vi "_SparkGetStatus.vi"(11 "SparkStatus":string="<SparkStatus>\n  <Autosampler>\n    <DeviceStatus>Standby</DeviceStatus>\n    <Detected>\n      <CanMixAndDilute>true</CanMixAndDilute>\n      <SerialNumber>000000</SerialNumber>\n      <FirmwareVersion>1.30</FirmwareVersion>\n      <PcbPartNumber>0840.604-03</PcbPartNumber>\n      <FpgaPartNumber>0840.141</FpgaPartNumber>\n      <FpgaVersion>2.10</FpgaVersion>\n      <FirmwarePartNumber>0840.100</FirmwarePartNumber>\n    </Detected>\n    <DetailedStatus>\n      <ActualTemperature>35</ActualTemperature>\n      <Setpoint>4</Setpoint>\n      <SamplePosition>NotAvailable</SamplePosition>\n      <Status>Standby</Status>\n      <InjectorPosition>Inject</InjectorPosition>\n      <IsVialMissing>false</IsVialMissing>\n      <PlatePosition>NotAvailable</PlatePosition>\n      <IsTemperatureControlOn>false</IsTemperatureControlOn>\n      <StatusCode>0</StatusCode>\n      <ErrorCode>0</ErrorCode>\n      <LastDCActionGuid>00000000-0000-0000-0000-000000000000</LastDCActionGuid>\n      <DoorOpenTime>0</DoorOpenTime>\n      <CommunicationErrorMessage />\n      <IsDoorOpen>false</IsDoorOpen>\n      <TrayType>Vials48</TrayType>\n      <Progress>0</Progress>\n    </DetailedStatus>\n    <LogCounters>\n      <InjectorValve>466</InjectorValve>\n      <IssA>0</IssA>\n      <SyringeValve>2569</SyringeValve>\n      <Syringe>3837</Syringe>\n    </LogCounters>\n    <AdvancedStatus>\n      <IssValvePosition>OneTwo</IssValvePosition>\n      <Valve1Out6Position>0</Valve1Out6Position>\n      <SSVPosition>Solvent1</SSVPosition>\n      <IsCompressorOn>false</IsCompressorOn>\n      <SyringeValvePosition>0</SyringeValvePosition>\n      <AdjustmentNeedleHorizontal>0</AdjustmentNeedleHorizontal>\n      <AdjustmentTray>0</AdjustmentTray>\n      <AdjustmentSyringe>0</AdjustmentSyringe>\n      <AdjustmentNeedleInEEprom>0</AdjustmentNeedleInEEprom>\n      <AdjustmentTrayInEEprom>0</AdjustmentTrayInEEprom>\n      <AdjustmentSyringeInEEprom>0</AdjustmentSyringeInEEprom>\n      <IsAux1On>false</IsAux1On>\n    </AdvancedStatus>\n    <Options>\n      <HasCooling>true</HasCooling>\n      <HasSSV>true</HasSSV>\n      <HasWashPort2>true</HasWashPort2>\n      <HasISSA>false</HasISSA>\n      <HasHeating>false</HasHeating>\n      <Has6PortValve>false</Has6PortValve>\n    </Options>\n    <Config>\n      <LoopVolume>100</LoopVolume>\n      <SyringeVolume>500</SyringeVolume>\n      <NeedleVolume>15</NeedleVolume>\n    </Config>\n  </Autosampler>\n  <ColumnOven>\n    <DeviceStatus>Standby</DeviceStatus>\n    <Detected>\n      <SerialNumber>130086</SerialNumber>\n      <FirmwareVersion>3.01</FirmwareVersion>\n      <PcbPartNumber>0886.603</PcbPartNumber>\n      <FpgaPartNumber>0886.104</FpgaPartNumber>\n      <FpgaVersion>1.00</FpgaVersion>\n      <FirmwarePartNumber>0886.105</FirmwarePartNumber>\n      <PcbVersion>03</PcbVersion>\n      <ColumnOvenOptions>\n        <HasCooling>false</HasCooling>\n        <HasColumnSwitcher>false</HasColumnSwitcher>\n      </ColumnOvenOptions>\n    </Detected>\n    <DetailedStatus>\n      <Status>Standby</Status>\n      <Setpoint>40</Setpoint>\n      <ActualTemperature>36</ActualTemperature>\n      <ActualValvePosition>0</ActualValvePosition>\n      <VapourAlarmSensitivity>Standard</VapourAlarmSensitivity>\n      <StatusCode>0</StatusCode>\n      <ErrorCode>0</ErrorCode>\n      <LastDCActionGuid>00000000-0000-0000-0000-000000000000</LastDCActionGuid>\n      <RequestSetpoint>0</RequestSetpoint>\n      <CustomCommandResponse />\n      <IsOvenOn>false</IsOvenOn>\n    </DetailedStatus>\n    <Service>\n      <IsInServiceMode>false</IsInServiceMode>\n      <ColumnSelectionHomeSensor>Unknown</ColumnSelectionHomeSensor>\n      <ColumnSelectionLegalSensor>Unknown</ColumnSelectionLegalSensor>\n      <HeaterFanSpeed>0</HeaterFanSpeed>\n    </Service>\n    <LogCounters>\n      <ColumnSwitch>0</ColumnSwitch>\n    </LogCounters>\n    <FlashStatus>\n      <Status>Ready</Status>\n      <StatusOfFlash>0</StatusOfFlash>\n      <Percentage>0</Percentage>\n      <Speed>0</Speed>\n    </FlashStatus>\n  </ColumnOven>\n  <LcPump>\n    <DeviceStatus>Running</DeviceStatus>\n    <DetectedA>\n      <SerialNumber>130060</SerialNumber>\n      <FirmwareVersion>1.14</FirmwareVersion>\n      <PcbPartNumber>0760.600-12</PcbPartNumber>\n      <FpgaPartNumber>0760.101</FpgaPartNumber>\n      <FpgaVersion>1.05</FpgaVersion>\n      <FirmwarePartNumber>0760.100</FirmwarePartNumber>\n    </DetectedA>\n    <DetectedB>\n      <SerialNumber>130060</SerialNumber>\n      <FirmwareVersion>1.14</FirmwareVersion>\n      <PcbPartNumber>0760.600-12</PcbPartNumber>\n      <FpgaPartNumber>0760.101</FpgaPartNumber>\n      <FpgaVersion>1.05</FpgaVersion>\n      <FirmwarePartNumber>0760.100</FirmwarePartNumber>\n    </DetectedB>\n    <DetailedStatus>\n      <Status>Standby</Status>\n      <ModuleA>\n        <ActualPressure>0</ActualPressure>\n        <Solvent>Solvent1</Solvent>\n        <ActualFlow>0</ActualFlow>\n        <Status>Standby</Status>\n        <MaxPressure>1240</MaxPressure>\n        <CompressibilityFactor>0</CompressibilityFactor>\n        <FlowCompensationFactor>0</FlowCompensationFactor>\n        <ProgrammedFlow>0</ProgrammedFlow>\n        <ErrorCode>0</ErrorCode>\n        <StatusCode>0</StatusCode>\n        <IsPumpOn>false</IsPumpOn>\n      </ModuleA>\n      <ModuleB>\n        <ActualPressure>0</ActualPressure>\n        <Solvent>Solvent1</Solvent>\n        <ActualFlow>0</ActualFlow>\n        <Status>Standby</Status>\n        <MaxPressure>1240</MaxPressure>\n        <CompressibilityFactor>0</CompressibilityFactor>\n        <FlowCompensationFactor>0</FlowCompensationFactor>\n        <ProgrammedFlow>0</ProgrammedFlow>\n        <ErrorCode>0</ErrorCode>\n        <StatusCode>0</StatusCode>\n        <IsPumpOn>false</IsPumpOn>\n      </ModuleB>\n      <IsDegasserOn>true</IsDegasserOn>\n      <LastDCActionGuid>00000000-0000-0000-0000-000000000000</LastDCActionGuid>\n    </DetailedStatus>\n    <ServiceA>\n      <Fan1Speed>0</Fan1Speed>\n      <Fan2Speed>0</Fan2Speed>\n      <IsInServiceMode>false</IsInServiceMode>\n    </ServiceA>\n    <ServiceB>\n      <Fan1Speed>0</Fan1Speed>\n      <Fan2Speed>0</Fan2Speed>\n      <IsInServiceMode>false</IsInServiceMode>\n    </ServiceB>\n    <LogCountersA>\n      <OperationTime>0</OperationTime>\n      <NumberOfRevolutions>0</NumberOfRevolutions>\n      <VolumeLeftSeal>0</VolumeLeftSeal>\n      <VolumeRightSeal>0</VolumeRightSeal>\n    </LogCountersA>\n    <LogCountersB>\n      <OperationTime>0</OperationTime>\n      <NumberOfRevolutions>0</NumberOfRevolutions>\n      <VolumeLeftSeal>0</VolumeLeftSeal>\n      <VolumeRightSeal>0</VolumeRightSeal>\n    </LogCountersB>\n  </LcPump>\n</SparkStatus>") -> (0 "PumpState":string, 1 "AS Status 2":string, 2 "LCStatus":string, 3 "Ready":bool, 4 "PumpB Status":string, 5 "Oven Status":string, 6 "PumpA Status":string, 7 "AS Status":string)   [LabVIEW 2015]
panel:
  out "OvenState":string
  out "ASState":string
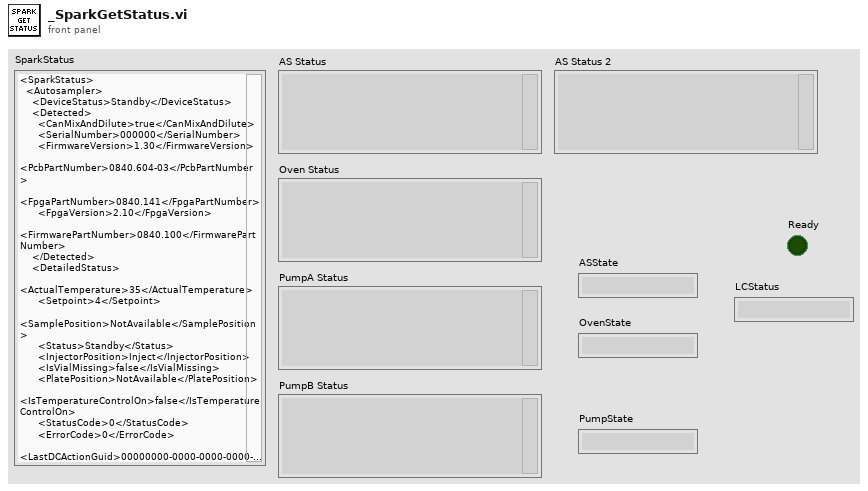
[diagram p1: front panel]
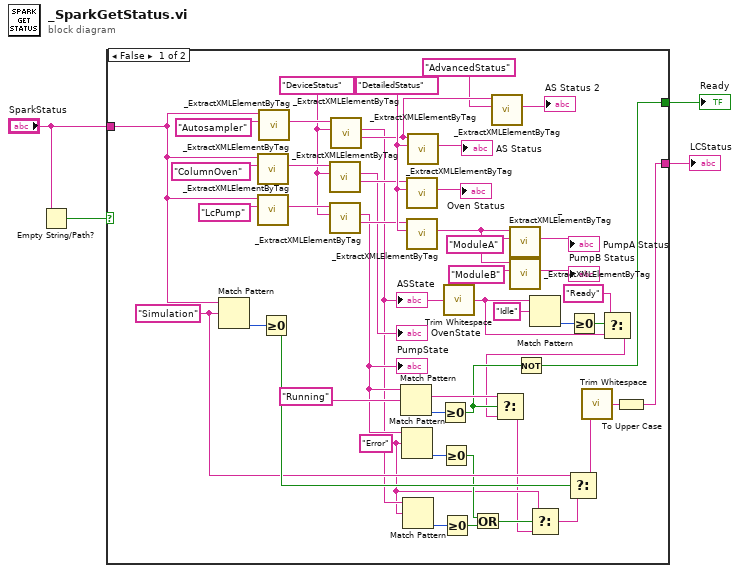
[diagram p0: block diagram]
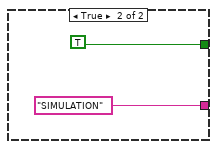
[diagram p2: hidden frame]
diagram:
  n1 = Empty String/Path?(string/path="SparkStatus") -> (empty?=w3:bool)
  n2 = case shown="False" w3 {
    tunnel: "SparkStatus" -> [w19 _]
    tunnel: [w14 "SIMULATION" ("y")] -> w2
    tunnel: [w31 TRUE] -> w1
    frame False {
      w17 = "Simulation" ("format string")
      w8 = "Error" ("regular expression")
      w47 = "DetailedStatus" ("TagName")
      w46 = "DeviceStatus" ("TagName")
      n3 = Match Pattern(string=w19, regular expression=w17) -> (offset past match=w20:i32)  [unwired: 4 out]
      n4 = call "_ExtractXMLElementByTag.vi"("TagName"="ColumnOven", "XML String"=w19) -> ("Element"=w49:string)  [unwired: 2 in, 3 out]
      n5 = call "_ExtractXMLElementByTag.vi"("TagName"="LcPump", "XML String"=w19) -> ("Element"=w48:string)  [unwired: 2 in, 3 out]
      n6 = call "_ExtractXMLElementByTag.vi"("TagName"="Autosampler", "XML String"=w19) -> ("Element"=w50:string)  [unwired: 2 in, 3 out]
      n7 = Greater Or Equal To 0?(x=w20) -> (x >= 0?=w18:bool)
      n8 = call "_ExtractXMLElementByTag.vi"("TagName"=w46, "XML String"=w49) -> ("TailingString"=w45:string, "Element"=→"OvenState":string)  [unwired: 2 in, 2 out]
      n9 = call "_ExtractXMLElementByTag.vi"("TagName"=w46, "XML String"=w48) -> ("TailingString"=w44:string, "Element"=w26:string)  [unwired: 2 in, 2 out]
      "PumpState" <- w26
      n10 = call "_ExtractXMLElementByTag.vi"("TagName"=w46, "XML String"=w50) -> ("TailingString"=w30:string, "Element"=w12:string)  [unwired: 2 in, 2 out]
      "ASState" <- w12
      n11 = Match Pattern(string=w26, regular expression="Running" ("search string/char (-)")) -> (match substring=w33:string, offset past match=w35:i32)  [unwired: 1 in, 2 out]
      n12 = Match Pattern(string=w26, regular expression=w8) -> (offset past match=w27:i32)  [unwired: 1 in, 3 out]
      n13 = Match Pattern(string=w12, regular expression=w8) -> (offset past match=w13:i32)  [unwired: 1 in, 3 out]
      n14 = call "_ExtractXMLElementByTag.vi"("TagName"=w47, "XML String"=w45) -> ("Element"=→"Oven Status":string)  [unwired: 2 in, 3 out]
      n15 = call "_ExtractXMLElementByTag.vi"("TagName"=w47, "XML String"=w44) -> ("Element"=w38:string)  [unwired: 2 in, 3 out]
      n16 = call "_ExtractXMLElementByTag.vi"("TagName"=w47, "XML String"=w30) -> ("Element"=→"AS Status":string)  [unwired: 2 in, 3 out]
      n17 = Greater Or Equal To 0?(x=w35) -> (x >= 0?=w32:bool)
      n18 = Greater Or Equal To 0?(x=w27) -> (x >= 0?=w10:bool)
      n19 = Greater Or Equal To 0?(x=w13) -> (x >= 0?=w11:bool)
      n20 = call <vilib>:"Trim Whitespace.vi"("string"=w12) -> ("trimmed string"=w21:string)  [unwired: 1 in]
      n21 = Or(x=w10, y=w11) -> (x .or. y?=w9:bool)
      n22 = call "_ExtractXMLElementByTag.vi"("TagName"="AdvancedStatus", "XML String"=w30) -> ("Element"=→"AS Status 2":string)  [unwired: 2 in, 3 out]
      n23 = call "_ExtractXMLElementByTag.vi"("TagName"="ModuleA", "XML String"=w38) -> ("Element"=→"PumpA Status":string)  [unwired: 2 in, 3 out]
      n24 = call "_ExtractXMLElementByTag.vi"("TagName"="ModuleB", "XML String"=w38) -> ("Element"=→"PumpB Status":string)  [unwired: 2 in, 3 out]
      n25 = Not(x=w32) -> (.not. x?=w31:bool)
      n26 = Match Pattern(string=w21, regular expression="Idle") -> (offset past match=w25:i32)  [unwired: 1 in, 3 out]
      n27 = Greater Or Equal To 0?(x=w25) -> (x >= 0?=w23:bool)
      n28 = Select(t="Ready" ("regular expression"), s=w23, f=w21) -> (s? t:f=w7:string)
      n29 = Select(t=w33, s=w32, f=w7) -> (s? t:f=w6:string)
      n30 = Select(t=w8, s=w9, f=w6) -> (s? t:f=w5:string)
      n31 = Select(t=w17, s=w18, f=w5) -> (s? t:f=w16:string)
      n32 = call <vilib>:"Trim Whitespace.vi"("string"=w16) -> ("trimmed string"=w15:string)  [unwired: 1 in]
      n33 = To Upper Case(1:w15) -> (0:w14:string)
    }
    frame True {
    }
  }
  "Ready" <- w1
  "LCStatus" <- w2
